vi "svl_Decimated Exp Avg Resampled Level (1 Ch).vi"(5 "time constant [ms]":dbl=125.0 format="%.2f", 6 "decimation factor":i32, 7 "exponential mode":enum16{"Slow", "Fast", "Impulse", "Custom"}(ring)=enum."Fast", 8 "error in (no error)":errorcluster, 9 "processing state":T1(ring), 11 "even angle signal":T2 {"even angle signal" format="%.2f"; "dr" format="%.2f"; "r0" format="%.2f"}) -> (0 "error out":errorcluster, 1 "actual time constant [ms]":dbl=125.0 format="%.2f", 3 "even angle signal":T2 {"even angle signal" format="%.2f"; "dr" format="%.2f"; "r0" format="%.2f"}, 4 "actual decimation factor":i32=1 min=1 step=1)   [LabVIEW 2017]
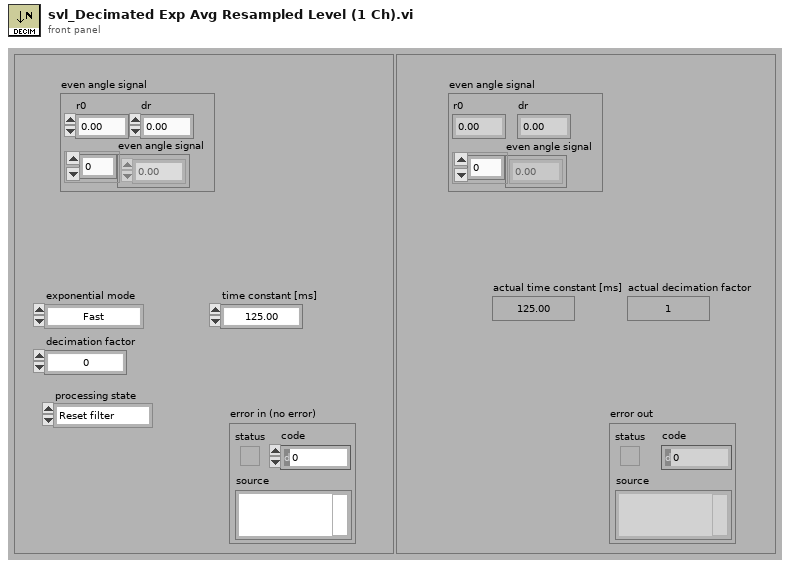
[diagram p1: front panel]
types:
  T1 = enum16{"Reset filter", "Restart averaging", "Continue processing"}
  T2 = cluster{"r0":dbl, "dr":dbl, "even angle signal":dbl[]}
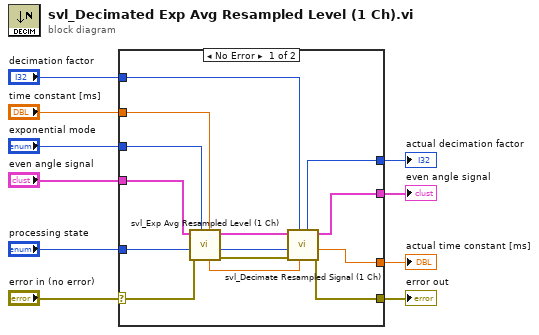
[diagram p0: block diagram]
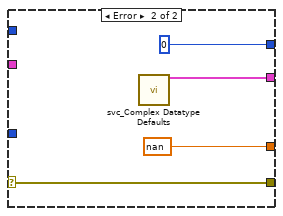
[diagram p2: hidden frame]
diagram:
  n1 = case shown="No Error" "error in (no error)" {
    selector: "error in (no error)" -> [w13 w27]
    tunnel: "even angle signal" -> [w11 _]
    tunnel: [w12 w27] -> w9
    tunnel: [w22 w25] -> w8
    tunnel: "exponential mode" -> [w21 _]
    tunnel: "decimation factor" -> [w20 _]
    tunnel: [w19 nan ("new dt")] -> w5
    tunnel: [w18 0 ("actual decimation factor")] -> w4
    tunnel: "time constant [ms]" -> [w17 _]
    tunnel: "processing state" -> [w16 _]
    frame No Error {
      n2 = call <vilib>:"svl_Exp Avg Resampled Level (1 Ch).vi"("timeConstant"=w17, "exponential mode"=w21, "error in (no error)"=w13, "processing state"=w16, "even angle signal"=w11) -> ("error out"=w24:errorcluster, "dup processing state"=w15:T1, "even angle signal"=w23:T2, "actual time constant [ms]"=w14:dbl)  [unwired: 3 in]
      n3 = call <vilib>:"svl_Decimate Resampled Signal (1 Ch).vi"("actual time constant [ms]"=w14, "decimation factor"=w20, "error in (no error)"=w24, "processing state"=w15, "even angle signal"=w23) -> ("error out"=w12:errorcluster, "dup actual time constant [ms]"=w19:dbl, "even angle signal"=w22:T2, "actual decimation factor"=w18:i32)  [unwired: 3 in]
    }
    frame Error {
      n4 = call <vilib>:"svc_Complex Datatype Defaults.vi"() -> ("empty spectrum"=w25:cluster{"f0":dbl, "df":dbl, "magnitude":dbl[]})  [unwired: 11 in, 8 out]
    }
  }
  "error out" <- w9
  "even angle signal" <- w8
  "actual time constant [ms]" <- w5
  "actual decimation factor" <- w4
